vi "niRFUtil LCAPI Copy 1D Array (5 DBL).vi"(0 "Source0 1D Array (DBL)":dbl[](array[numeric]) format="%.2f", 5 "Source1 1D Array (DBL)":dbl[](array[numeric]) format="%.2f", 7 "Source2 1D Array (DBL)":dbl[](array[numeric]) format="%.2f", 9 "Source3 1D Array (DBL)":dbl[](array[numeric]) format="%.2f", 11 "error in (no error)":errorcluster, 12 "Data Copy Descriptor":u64, 13 "Source4 1D Array (DBL)":dbl[](array[numeric]) format="%.2f") -> (3 "Source4 Out":dbl[](array[numeric]) format="%.2f", 4 "Source0 Out":dbl[](array[numeric]) format="%.2f", 6 "Source1 Out":dbl[](array[numeric]) format="%.2f", 8 "Source2 Out":dbl[](array[numeric]) format="%.2f", 10 "Source3 Out":dbl[](array[numeric]) format="%.2f", 15 "error out":errorcluster)   [LabVIEW 2015, in "niRFUtil.lvlib"]
uses:
  niRFUtil.lvlib
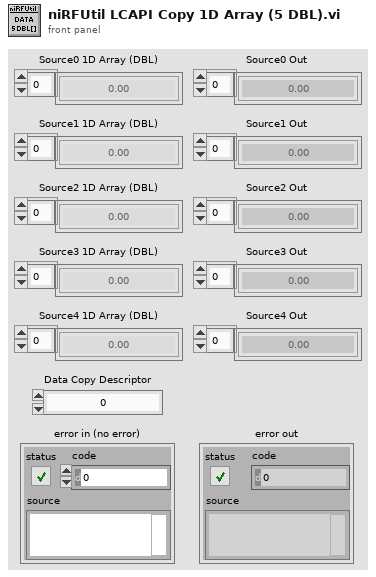
[diagram p1: front panel]
types:
  T1 = cluster{"status":bool, "return type":i32, "errorString":string}
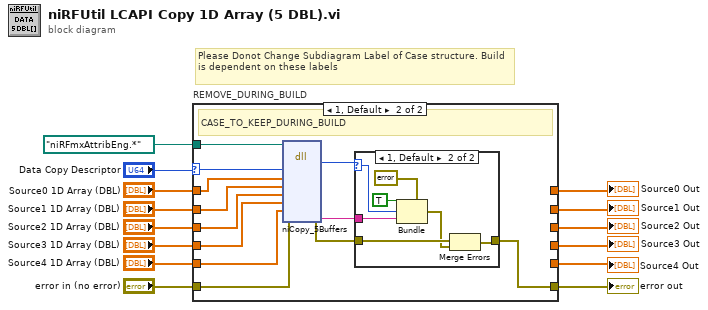
[diagram p0: block diagram]
diagram:
  # "Please Donot Change Subdiagram Label of Case structure. Build is dependent on these labels"
  n1 = case "REMOVE_DURING_BUILD" shown="1, Default" "Data Copy Descriptor" {
    selector: "Data Copy Descriptor" -> [_ w22]
    tunnel: [w20 w32] -> w14
    tunnel: "error in (no error)" -> [w20 w31]
    tunnel: "Source1 1D Array (DBL)" -> [w16 w30]
    tunnel: "Source2 1D Array (DBL)" -> [w17 w29]
    tunnel: "Source3 1D Array (DBL)" -> [w18 w28]
    tunnel: "Source4 1D Array (DBL)" -> [w19 w27]
    tunnel: "Source0 1D Array (DBL)" -> [w15 w26]
    tunnel: [w19 _] -> w6
    tunnel: [w18 _] -> w5
    tunnel: [w17 _] -> w4
    tunnel: [w16 _] -> w3
    tunnel: [w15 _] -> w2
    tunnel: path "niRFmxAttribEng.*" ("path in") -> [_ w21]
    frame 0 {
      # "Development"
    }
    frame 1, Default {
      # "CASE_TO_KEEP_DURING_BUILD"
      n2 = dll-call lib="niRFmxAttribEng.*" fn="niCopy_5Buffers"(path in=w21, error in=w31, "dataCopyDescriptor"=w22, "source0"=w26, "source1"=w30, "source2"=w29, "source3"=w28, "source4"=w27) -> (error out=w23:errorcluster, "return type"=w25:i32, "errorString"=w24:string)  [unwired: 8 in, 1 out]
      n3 = case shown="1, Default" w25 {
        selector: w25 -> [_ w39]
        tunnel: w24 -> [_ w38]
        tunnel: w23 -> [w33 w36]
        tunnel: [w33 w37] -> w32
        frame 0 {
        }
        frame 1, Default {
          n4 = Bundle(cluster=T1 {"status"=FALSE, "return type"=0, "errorString"=""}, "status"=TRUE, "return type"=w39, "errorString"=w38) -> (w35:T1)
          n5 = Merge Errors(w36, w35) -> (w37:errorcluster)
        }
      }
    }
  }
  "error out" <- w14
  "Source0 Out" <- w2
  "Source1 Out" <- w3
  "Source2 Out" <- w4
  "Source3 Out" <- w5
  "Source4 Out" <- w6
